vi "CH_LM Config Trigger Bus Control.vi"(0 "Meter Index":i32, 2 "Trigger Bus Control (2)":T1=enum."Independent", 5 "error in (no error)":errorcluster, 7 "Timeout / ms (3000)":i32=3000, 8 "Action (query)":bool, 9 "Lock Timeout / ms (1000)":i32=1000) -> (11 "Lock timed out":bool, 14 "Meter Index":i32, 16 "Trigger Bus Control":T1=enum."Independent", 19 "error out":errorcluster)   [LabVIEW 2012, in "CH_LM.lvlib"]
doc: "This command will set/query the trigger bus direction."
uses:
  CH_LM.lvlib
  CH_LM Trigger Bus Control.ctl
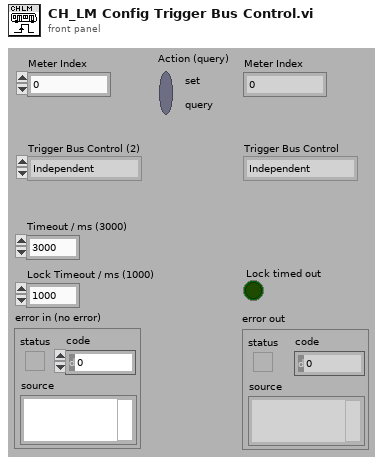
[diagram p1: front panel]
types:
  T1 = typedef "CH_LM.lvlib/CH_LM Trigger Bus Control.ctl" = enum16{"Host", "Guest", "Independent"}
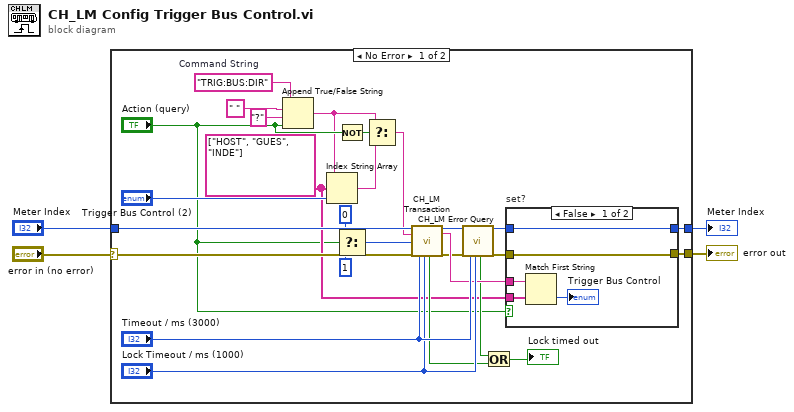
[diagram p0: block diagram]
diagram:
  n1 = case shown="No Error" "error in (no error)" {
    selector: "error in (no error)" -> [w31 w40]
    tunnel: [w29 w40] -> w4
    tunnel: "Meter Index" -> [w30 w39]
    tunnel: [w28 w39] -> w1
    frame No Error {
      w10 = string[] ["HOST", "GUES", "INDE"] ("string array")
      w25 = "TRIG:BUS:DIR"  # Command String
      n2 = Append True/False String(1:"Action (query)", 2:"?" ("true string"), 3:" ", 4:w25) -> (0:w7:string)
      n3 = Index String Array(1:"Trigger Bus Control (2)", 2:w10, 3:w7) -> (0:w6:string)
      n4 = Not(x="Action (query)") -> (.not. x?=w8:bool)
      n5 = Select(t=0, s="Action (query)", f=1 ("NofStrings (-1:all)")) -> (s? t:f=w21:i32)
      n6 = Select(t=w7, s=w8, f=w6) -> (s? t:f=w5:string)
      n7 = call "CH_LM Transaction.vi"("Meter Index"=w30, "Command String"=w5, "NofStrings (-1:all)"=w21, "error in (no error)"=w31, "Timeout / ms (3000)"="Timeout / ms (3000)", "Lock Timeout / ms (1000)"="Lock Timeout / ms (1000)") -> ("Lock timed out"=w14:bool, "Meter Index"=w19:i32, "Response"=w24:string, "error out"=w17:errorcluster)  [unwired: 10 out]
      n8 = call "CH_LM Error Query.vi"("Meter Index"=w19, "error in (no error)"=w17, "Timeout / ms (3000)"="Timeout / ms (3000)", "Lock Timeout / ms (1000)"="Lock Timeout / ms (1000)") -> ("Lock timed out"=w15:bool, "Meter Index"=w18:i32, "error out"=w16:errorcluster)  [unwired: 13 out]
      n9 = Or(x=w15, y=w14) -> (x .or. y?=→"Lock timed out":bool)
      n10 = case "set?" shown="False" "Action (query)" {
        tunnel: w24 -> [w35 _]
        tunnel: w16 -> [w34 w38]
        tunnel: [w34 w38] -> w29
        tunnel: w18 -> [w36 w37]
        tunnel: [w36 w37] -> w28
        tunnel: w10 -> [w32 _]
        frame False {
          n11 = Match First String(2:w32, 3:w35) -> (0:→"Trigger Bus Control":i32)  [unwired: 1 out]
        }
        frame True {
        }
      }
    }
    frame Error {
    }
  }
  "error out" <- w4
  "Meter Index" <- w1
